vi "Actor Core.vi"(8 "error in":errorcluster, 11 "IViewable In":refnum<class "IViewable.lvclass">) -> (0 "error out":errorcluster, 3 "Actor out":refnum<class "Actor.lvclass">)   [LabVIEW 2015, in "IViewable.lvlib" / "IViewable.lvclass"]
doc: "(<B>Filename</B>: Actor Framework.lvlib:Actor.lvclass:Actor Core.vi)\n\nReceives messages to the actor, reacts to them, and initiates any error handling that may shut the actor down.\n\nDescendant classes may override this VI to append parallel tasks for the actor to complete while it handles messages. Overrides use the Call Parent Method node."
uses:
  IViewable.lvclass
  <vilib>/ActorFramework/Actor/Actor.lvclass
  AutoRegistration/AutoEventActor/AutoEventActor.lvclass
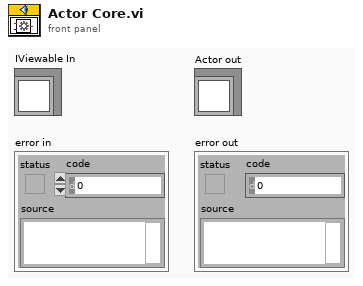
[diagram p1: front panel]
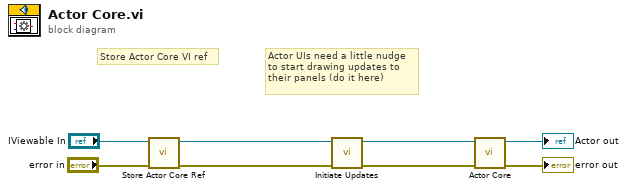
[diagram p0: block diagram]
diagram:
  # "Actor UIs need a little nudge\nto start drawing updates to \ntheir panels (do it here)"
  # "Store Actor Core VI ref"
  n1 = call "Store Actor Core Ref.vi"("error in (no error)"="error in", "IViewable In"="IViewable In") -> ("error out"=w6:errorcluster, "IViewable Out"=w3:refnum<class "IViewable.lvclass">)  [unwired: 8 in]
  n2 = call-dynamic "Initiate Updates.vi"("error in (no error)"=w6, "IViewable In"=w3) -> ("error out"=w2:errorcluster, "IViewable Out"=w1:refnum<class "IViewable.lvclass">)  [unwired: 8 in]
  n3 = call-parent "Actor Core.vi"("error in"=w2, "Actor in"=w1) -> ("error out"=→"error out":errorcluster, "Actor out"=→"Actor out":refnum<class "Actor.lvclass">)  [unwired: 8 in]
